vi "_API_BINANCE_GET_AccountSnapshot.vi"(0 "BinanceAPI in":refnum<class "BinanceAPI_.lvclass">, 5 "AccountSnapshot":T2={"type"=enum."MARGIN", "startTime"=0, "endTime"=0, "limit"=0, "recvWindow"=0}, 11 "error in (no error)":errorcluster) -> (4 "BinanceAPI out":refnum<class "BinanceAPI_.lvclass">, 6 "type and defaults":T1, 14 "Dane":string, 15 "error out":errorcluster)   [LabVIEW 2022 SP3, in "BinanceAPI_.lvclass"]
doc: "https://binance-docs.github.io/apidocs/spot/en/#daily-account-snapshot-user_data"
uses:
  BinanceAPI_.lvclass
  BinanceAPI_.lvclass/BinanceAPI_.ctl
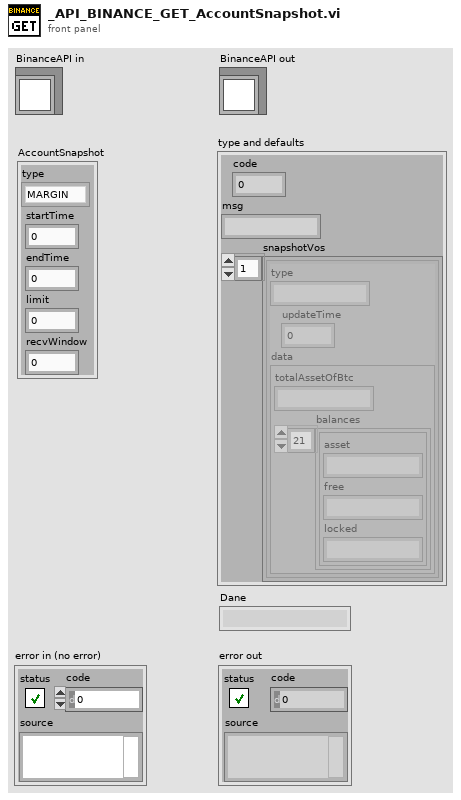
[diagram p1: front panel]
types:
  T1 = cluster{"code":dbl, "msg":string, "snapshotVos":cluster{"type":string, "updateTime":dbl, "data":cluster{"totalAssetOfBtc":string, "balances":cluster{"asset":string, "free":string, "locked":string}[]}}[]}
  T2 = cluster{"type":enum16{"SPOT", "MARGIN", "FUTURES"}, "startTime":i32, "endTime":i32, "limit":i16, "recvWindow":i32}
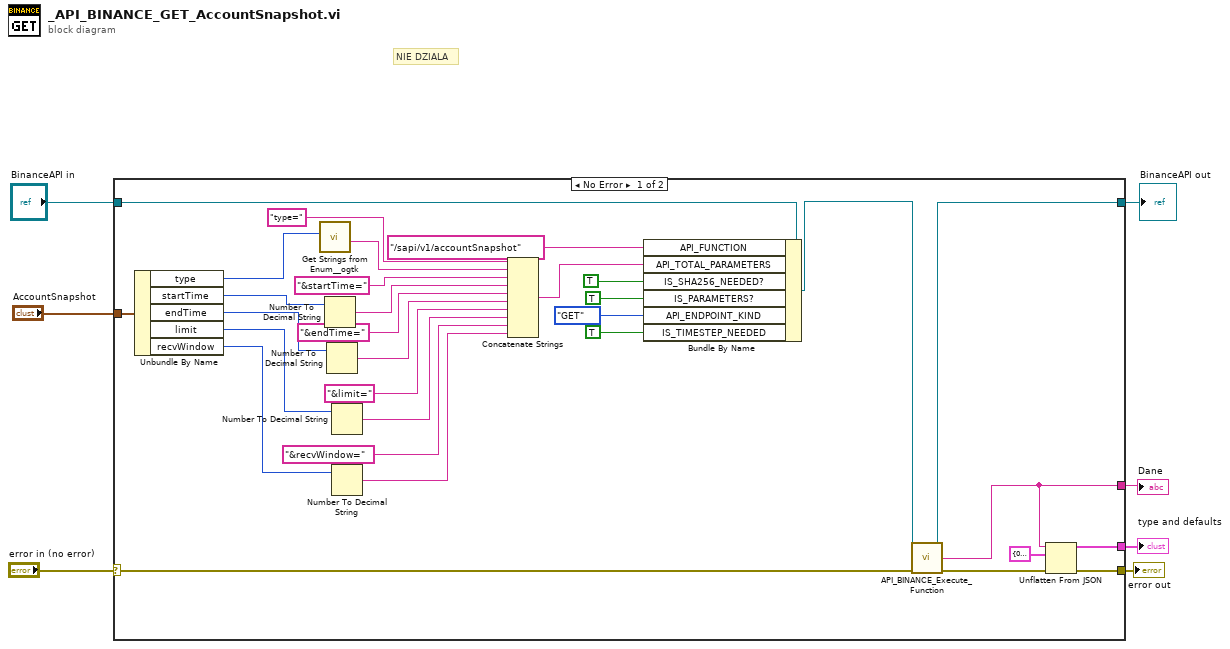
[diagram p0: block diagram]
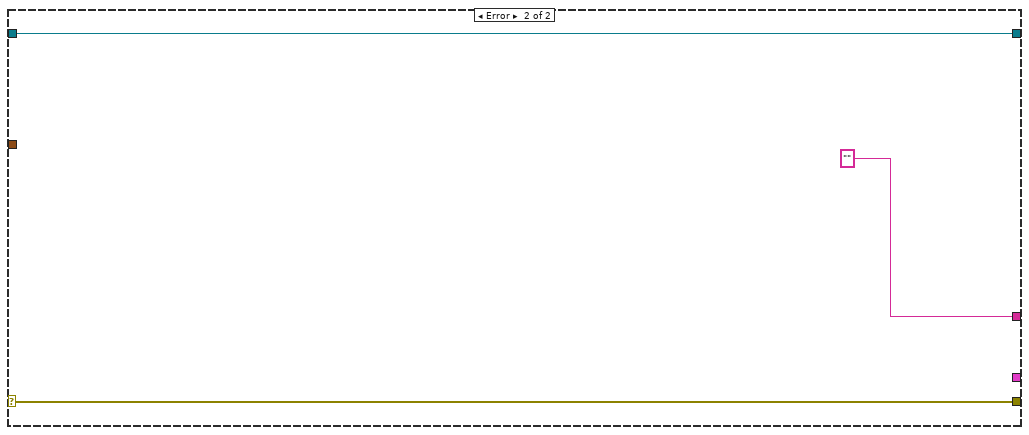
[diagram p2: hidden frame]
diagram:
  # "NIE DZIALA"
  n1 = case shown="No Error" "error in (no error)" {
    selector: "error in (no error)" -> [w14 w41]
    tunnel: [w11 w41] -> w6
    tunnel: [w15 w40] -> w1
    tunnel: "BinanceAPI in" -> [w17 w40]
    tunnel: "AccountSnapshot" -> [w34 _]
    tunnel: [w10 "" ("Dane")] -> w4
    tunnel: [w8 _] -> w3
    frame No Error {
      n2 = Unbundle By Name(w34) -> ("type"=w19:enum16{"SPOT", "MARGIN", "FUTURES"}, "startTime"=w31:i32, "endTime"=w30:i32, "limit"=w28:i16, "recvWindow"=w29:i32)
      n3 = call <userlib>:"Get Strings from Enum__ogtk.vi"("Enum"=w19) -> ("String Value"=w13:string)  [unwired: 7 in, 3 out]
      n4 = Number To Decimal String(number=w31) -> (decimal integer string=w26:string)  [unwired: 1 in]
      n5 = Number To Decimal String(number=w30) -> (decimal integer string=w24:string)  [unwired: 1 in]
      n6 = Number To Decimal String(number=w28) -> (decimal integer string=w22:string)  [unwired: 1 in]
      n7 = Number To Decimal String(number=w29) -> (decimal integer string=w20:string)  [unwired: 1 in]
      n8 = Concatenate Strings("type=" ("API_FUNCTION 2"), w13, "&startTime=" ("API_FUNCTION 2"), w26, "&endTime=" ("API_FUNCTION 2"), w24, "&limit=" ("API_FUNCTION 2"), w22, "&recvWindow=" ("API_FUNCTION 2"), w20) -> (w35:string)
      n9 = Bundle By Name(cluster=w17, "API_FUNCTION"="/sapi/v1/accountSnapshot", "API_TOTAL_PARAMETERS"=w35, "IS_SHA256_NEEDED?"=TRUE, "IS_PARAMETERS?"=TRUE, "API_ENDPOINT_KIND"=enum16{"POST", "DELETE", "GET", "PUT"}."GET", "IS_TIMESTEP_NEEDED"=TRUE) -> (w16:refnum<class "BinanceAPI_.lvclass">)
      n10 = call "API_BINANCE_Execute_Function.vi"("BinanceAPI in"=w16, "error in (no error)"=w14) -> ("BinanceAPI out"=w15:refnum<class "BinanceAPI_.lvclass">, "Body"=w10:string, "error out"=w12:errorcluster)  [unwired: 9 in, 2 out]
      n11 = Unflatten From JSON(JSON string=w10, type and defaults=T1 {"code"=0.0, "msg"="", "snapshotVos"=[]}, error in (no error)=w12) -> (value=w8:T1, error out=w11:errorcluster)  [unwired: 4 in]
    }
    frame Error {
    }
  }
  "error out" <- w6
  "Dane" <- w4
  "type and defaults" <- w3
  "BinanceAPI out" <- w1
